vi "Comm_FileSave.vi"(7 "Console":refnum<vi>, 8 "error in (no error)":errorcluster, 9 "Code":string, 10 "Console In":string, 11 "Python":T1) -> (0 "error out":errorcluster, 2 "Console":string, 3 "Python":T1)   [LabVIEW 2024]
uses:
  PythonCtrl.ctl
  Processors.ctl
  <vilib>/Utility/error.llb/Trim Whitespace One-Sided.vi
panel:
  out "File sent":string[](array[string])
  out "Array":u32[](array[numeric])
  out "replies":string[](array[string])
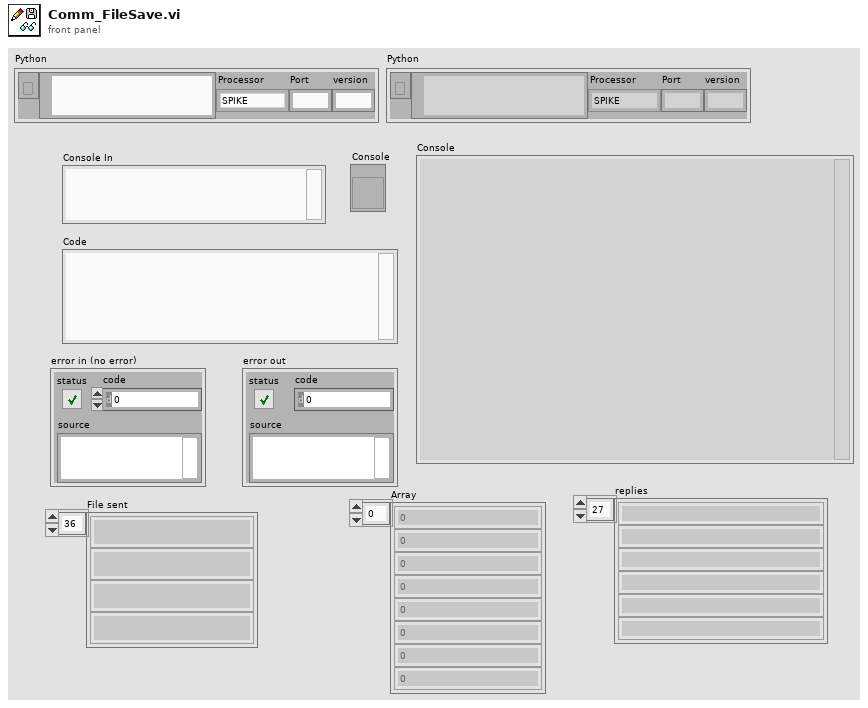
[diagram p1: front panel]
types:
  T1 = typedef "PythonCtrl.ctl" = cluster{"session":refnum<k35>, "PyPath":path, "Processor":T2, "Port":string, "version":string}
  T2 = typedef "Processors.ctl" = enum16{"SPIKE", "Pi", "Pi_ssh", "OpenMV", "Dunio"}
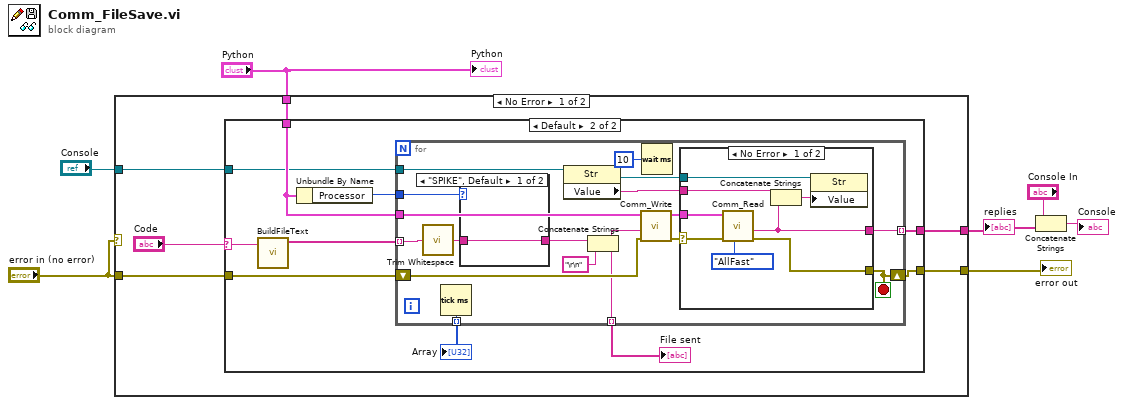
[diagram p0: block diagram]
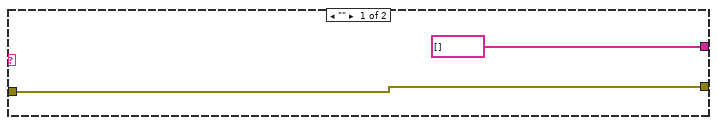
[diagram p2: hidden frame]
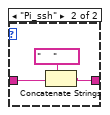
[diagram p3: hidden frame]
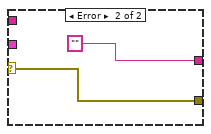
[diagram p4: hidden frame]
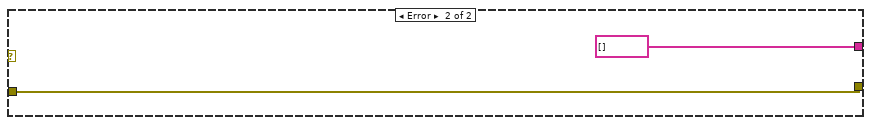
[diagram p5: hidden frame]
diagram:
  n1 = case shown="No Error" "error in (no error)" {
    tunnel: [w13 w57] -> w7
    tunnel: [w12 string[] []] -> w5
    tunnel: "Python" -> [w11 _]
    tunnel: "error in (no error)" -> [w10 w57]
    tunnel: "Console" -> [w9 _]
    frame No Error {
      n2 = case shown="Default" "Code" {
        selector: "Code" -> [_ w18]
        tunnel: [w15 w25] -> w13
        tunnel: [string[] [] w24] -> w12
        tunnel: w11 -> [_ w23]
        tunnel: w10 -> [w15 w20]
        tunnel: w9 -> [_ w21]
        frame "" {
        }
        frame Default {
          n3 = call "BuildFileText.vi"("Code"=w18) -> ("commands"=w19:string[])  [unwired: 9 in, 1 out]
          n4 = Unbundle By Name(w23) -> ("Processor"=w17:T2)
          n5 = for {
            tunnel: w23 -> [w30]
            tunnel: [w39] -> w24 mode=indexing
            shift-right: [w38] -> w25
            shift-left: w20 -> [w41]
            tunnel: [w37] -> w22 mode=indexing
            tunnel: w21 -> [w36]
            tunnel: w19 -> [w31] mode=indexing
            tunnel: w17 -> [w29]
            tunnel: [w26] -> w16 mode=indexing
            stop <- w38 stop-if-true
            n6 = call <vilib>:"Trim Whitespace.vi"("string"=w31) -> ("trimmed string"=w27:string)  [unwired: 1 in]
            n7 = Tick Count (ms)() -> (millisecond timer value=w37:u32)
            n8 = case shown="\"SPIKE\", Default" w29 {
              tunnel: [w42 w43] -> w28
              tunnel: w27 -> [w42 w45]
              frame "SPIKE", Default {
              }
              frame "Pi_ssh" {
                n9 = Concatenate Strings("    " ("delimiter (Tab)"), w45) -> (w43:string)
              }
            }
            n10 = property class="Str"(reference=w36) -> (reference out=w34:refnum<vi>, "Value"=w35:string)  [unwired: 1 in, 1 out]
            n11 = Concatenate Strings(w28, "\r\n" ("delimiter (Tab)")) -> (w26:string)
            n12 = call "Comm_Write.vi"("error in (no error)"=w41, "Text to write"=w26, "Python"=w30) -> ("error out"=w40:errorcluster)  [unwired: 7 in, 1 out]
            n13 = Wait (ms)(milliseconds to wait=u32 10) -> ()  [unwired: 1 out]
            n14 = case shown="No Error" w40 {
              selector: w40 -> [w51 w54]
              tunnel: [w53 w54] -> w38
              tunnel: [w49 ""] -> w39
              tunnel: w30 -> [w52 _]
              tunnel: w35 -> [w50 _]
              tunnel: w34 -> [w48 _]
              frame No Error {
                n15 = call "Comm_Read.vi"("Task"=enum16{"Instant", "All", "AllFast", "Params"}."AllFast", "error in (no error)"=w51, "Python"=w52) -> ("error out"=w53:errorcluster, "Text read"=w49:string)  [unwired: 7 in]
                n16 = Concatenate Strings(w50, w49) -> (w47:string)
                n17 = property class="Str"(reference=w48, "Value"=w47) -> ()  [unwired: 1 in, 2 out]
              }
              frame Error {
              }
            }
          }
          "Array" <- w22
          "File sent" <- w16
        }
      }
    }
    frame Error {
    }
  }
  "error out" <- w7
  "replies" <- w5
  n18 = Concatenate Strings("Console In", w5) -> (→"Console":string)
  "Python" <- "Python"
